vi "InitTableFromDevices.vi"(6 "Defer Updates? (T)":bool=TRUE, 7 "Layout Ref":refnum<vi>, 8 "error in (no error)":errorcluster, 10 "Table Ref in":refnum<vi>, 11 "Devices queue":refnum<queue>) -> (0 "error out":errorcluster, 1 "Col array":refnum<class "Column.lvclass">[](array[class]), 2 "DevNums":i32[](array[numeric]), 3 "Devices queue out":refnum<queue>)   [LabVIEW 2013]
doc: "Initialize SetList Table from Device array. \"DevNums\" and \"Col array\" are output and must be set. Devices out only needs to be set if \"Devices in\" is empty.\n\nIf \"Devices in\" is empty, a master object (PulseBlaster) is initialized with a single row of default data and the \"default layout\" is added to the Layout ring. If \"Devices in\" is not empty, it is up to the programmer to make sure Layouts match the devices.\n\nEvidently, this VI needs write access to the Column array."
uses:
  ColumnVIs/Column/Column.lvclass
  Device/Device.lvclass
  Pulseblaster/Pulseblaster.lvclass
  Master Device/Master Device.lvclass
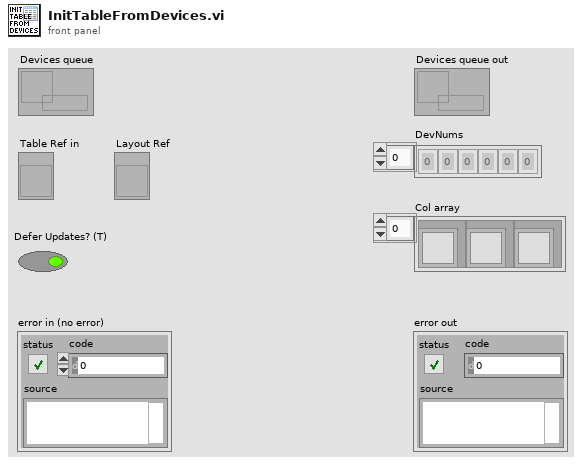
[diagram p1: front panel]
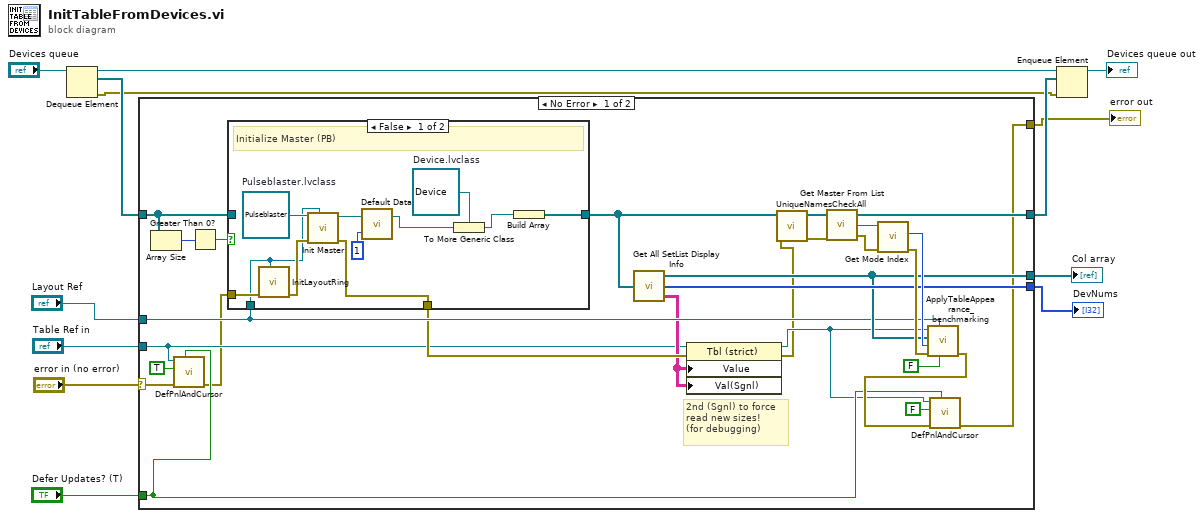
[diagram p0: block diagram]
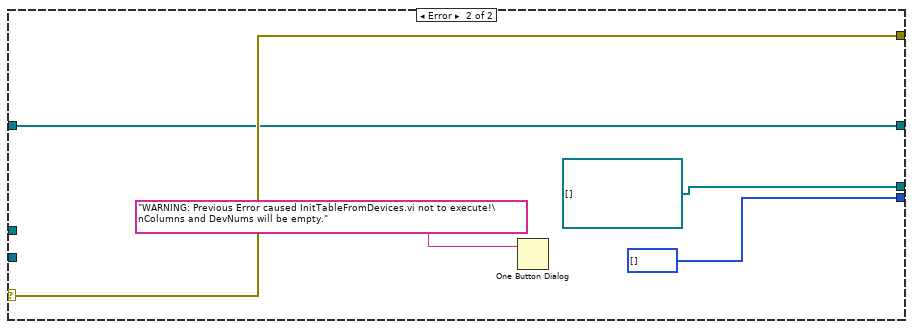
[diagram p3: hidden frame]
diagram:
  n1 = Dequeue Element(queue="Devices queue") -> (queue out=w7:refnum<queue>, element=w4:refnum<class "Device.lvclass">[], error out=w1:errorcluster)  [unwired: 2 in, 1 out]
  n2 = case shown="No Error" "error in (no error)" {
    selector: "error in (no error)" -> [w23 w58]
    tunnel: [w25 w58] -> w2
    tunnel: "Table Ref in" -> [w22 _]
    tunnel: "Defer Updates? (T)" -> [w20 _]
    tunnel: w4 -> [w40 w54]
    tunnel: [w39 w54] -> w5
    tunnel: [w34 i32[] [] ("DevNums")] -> w11
    tunnel: [w33 refnum<class "Column.lvclass">[] [] ("Columns")] -> w10
    tunnel: "Layout Ref" -> [w30 _]
    frame No Error {
      # "2nd (Sgnl) to force\nread new sizes!\n(for debugging)"
      n3 = Array Size(array=w40) -> (size(s)=w32:i32)
      n4 = call "DefPnlAndCursor.vi"("AllowDefPan? (T)"=w20, "error in (no error)"=w23, "DeferPanUpdts?"=TRUE, "Tbl Ctrl Refnum"=w22) -> ("error out"=w19:errorcluster)  [unwired: 7 in]
      n5 = Greater Than 0?(x=w32) -> (x > 0?=w31:bool)
      n6 = case shown="False" w31 {
        tunnel: w40 -> [_ w53]
        tunnel: [w46 w53] -> w17
        tunnel: w19 -> [w51 w52]
        tunnel: w30 -> [w41 _]
        tunnel: [w45 w52] -> w29
        frame False {
          w42 = refnum<class "Device.lvclass"> refnum  # Device.lvclass
          w50 = refnum<class "Pulseblaster.lvclass"> refnum  # Pulseblaster.lvclass
          # "Initialize Master (PB)"
          n7 = call "InitLayoutRing.vi"("Layouts Ring Refnum"=w41, "error in (no error)"=w51) -> ("error out"=w49:errorcluster)  [unwired: 9 in]
          n8 = call-dynamic "Init Master.vi"("Select Layout"=w41, "error in (no error)"=w49, "Pulseblaster in"=w50) -> ("error out"=w45:errorcluster, "Pulseblaster out"=w48:refnum<class "Pulseblaster.lvclass">)  [unwired: 7 in]
          n9 = call-dynamic "Default Data.vi"("Num Rows"=1, "Pulseblaster in"=w48) -> ("Pulseblaster out"=w44:refnum<class "Pulseblaster.lvclass">)  [unwired: 1 out]
          n10 = To More Generic Class(target class=w42, reference=w44) -> (generic class reference=w43:refnum<class "Device.lvclass">)
          n11 = Build Array(w43) -> (w46:refnum<class "Device.lvclass">[])
        }
        frame True {
          # "Device array has elements"
        }
      }
      n12 = call "Get All SetList Display Info.vi"("Devices"=w17) -> ("Columns"=w33:refnum<class "Column.lvclass">[], "DevNums"=w34:i32[], "Table Data"=w28:string[][])
      n13 = property on="Property Node" class="Tbl (strict)"(reference=w22, error in=w29, "Value"=w28, "Val(Sgnl)"=w28) -> (reference out=w18:refnum<vi>, error out=w15:errorcluster)
      n14 = call "UniqueNamesCheckAll.vi"("error in (no error)"=w15, "Devices"=w17) -> ("error out"=w14:errorcluster, "Devices out"=w16:refnum<class "Device.lvclass">[])  [unwired: 8 in]
      n15 = call "Get Master From List.vi"("error in"=w14, "Device List in"=w16) -> ("error out"=w37:errorcluster, "Master Device"=w38:refnum<class "Master Device.lvclass">, "Device List out"=w39:refnum<class "Device.lvclass">[])  [unwired: 1 in]
      n16 = call-dynamic "Get Mode Index.vi"("error in (no error)"=w37, "Master Device in"=w38) -> ("error out"=w36:errorcluster, "Mode Col"=w35:i32)  [unwired: 7 in, 1 out]
      n17 = call "ApplyTableAppearance_benchmarking.vi"("Defer Updates? (T)"=FALSE, "Layout Ring Ref"=w30, "error in (no error)"=w36, "Mode Index"=w35, "Col Array in"=w33, "Table Ref in"=w18) -> ("error out"=w26:errorcluster)  [unwired: 4 in, 1 out]
      n18 = call "DefPnlAndCursor.vi"("AllowDefPan? (T)"=w20, "error in (no error)"=w26, "DeferPanUpdts?"=FALSE, "Tbl Ctrl Refnum"=w18) -> ("error out"=w25:errorcluster)  [unwired: 7 in]
    }
    frame Error {
      n19 = One Button Dialog(message="WARNING: Previous Error caused InitTableFromDevices.vi not to execute!\nColumns and DevNums will be empty.") -> ()  [unwired: 1 in, 1 out]
    }
  }
  "error out" <- w2
  "DevNums" <- w11
  "Col array" <- w10
  n20 = Enqueue Element(queue=w7, element=w5, error in (no error)=w1) -> (queue out=→"Devices queue out":refnum<queue>)  [unwired: 1 in, 2 out]
